vi "OfeliaPressure.vi"() -> ()   [LabVIEW 2017]
uses:
  <vilib>/Platform/TimedLoop/XDataNode/timing_clust.ctl
  <vilib>/Platform/TimedLoop/XDataNode/nitl_modes.ctl
  <vilib>/Platform/TimedLoop/XDataNode/wakeup.ctl
  <vilib>/Instr/_visa.llb/VISA Configure Serial Port (Instr).vi
  <vilib>/platform/TimedLoop/XDataNode/XDataNode.xnode
  <vilib>/Platform/TimedLoop/XDataNode/XDNodeRunTimeDep.lvlib
panel:
  in  "Initial":dbl
  in  "Period":i64
  out "Final Pressure S":dbl
  out "In Range?":bool
  in  "T-Ramp\nTarget Pressure (Bar) S":dbl=0.01
  out "error out 5":errorcluster
  in  "T-Ramp Slow":bool
  out "Waveform Chart":dbl(graph)
  out "Final Pressure":dbl
  in  "S-Ramps\nTarget Pressure (Bar)":dbl
  in  "T-Ramp":bool
  in  "S-Ramp":bool
  out "error out 4":errorcluster
  out "In Range?":bool
  out "error out 3":errorcluster
  in  "ZERO":bool
  out "Final Pressure":dbl
  out "Ramp Rate\nFinal Value":dbl
  out "In Range?":bool
  in  "T-Ramp\nTarget Pressure (Bar)":dbl=0.01
  out "error out 2":errorcluster
  in  "Step 2":bool
  out "In Range?":bool
  in  "Ramp Rate":dbl=0.01
  in  "Step 1":bool
  in  "Stop":bool
  in  "VISA resource name":refnum<visa-resource-name>="COM1"
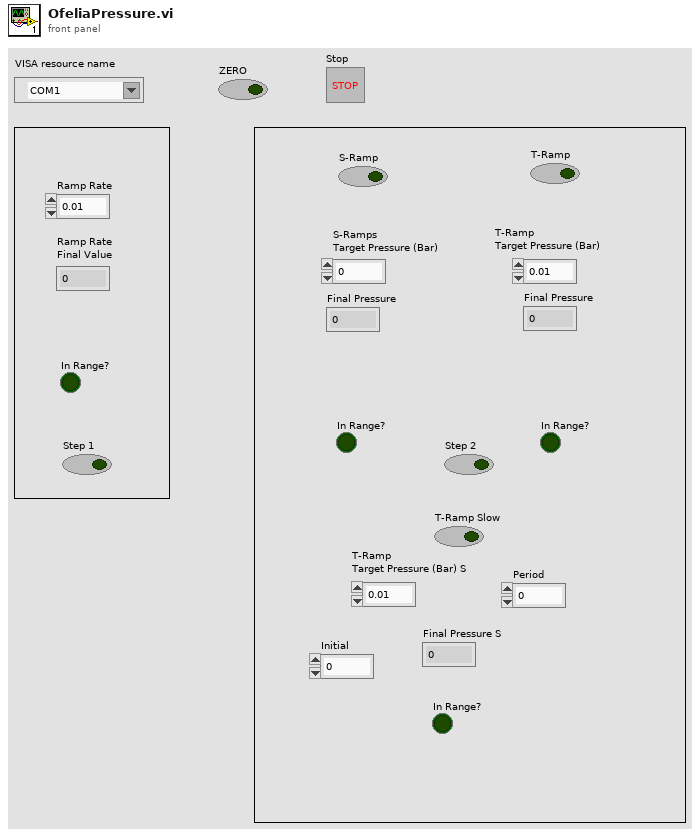
[diagram p1: front panel]
types:
  T1 = typedef "XDNodeRunTimeDep.lvlib/timing_clust.ctl" = cluster{"Expected End [f-1]":u64, "Actual End [f-1]":u64, "Finished Late? [f-1]":bool, "Expected End [i-1]":u64, "Actual End [i-1]":u64, "Finished Late? [i-1]":bool, "Expected Start [i]":u64, "Actual Start [i]":u64, "Expected Start [f]":u64, "Actual Start [f]":u64, "Source Name":string, "Structure Name":string, "Period":i64, "Deadline":i64, "Offset":i64, "Start":i64, "Priority":i32, "Timeout":i32, "Mode":T2, "Wakeup Reason":T3, "Error":errorcluster, "Source Type":string, "Secondary Source Type":string, "Global End Time":u64, "Global Start Time":u64, "Frame Duration":u64, "Iteration Duration":u64, "Assigned CPU":i32, "I/O Scan Engine Mode":u32}
  T2 = typedef "XDNodeRunTimeDep.lvlib/nitl_modes.ctl" = enum32{"No Change", "Process missed periods, maintain original phase", "Discard missed periods, maintain original phase", "Process missed periods, ignore original phase", "Discard missed periods, ignore original phase"}
  T3 = typedef "XDNodeRunTimeDep.lvlib/wakeup.ctl" = enum32{"Normal", "Aborted", "Asynchronous wakeup", "Timing source error", "Timed loop error", "Timeout"}
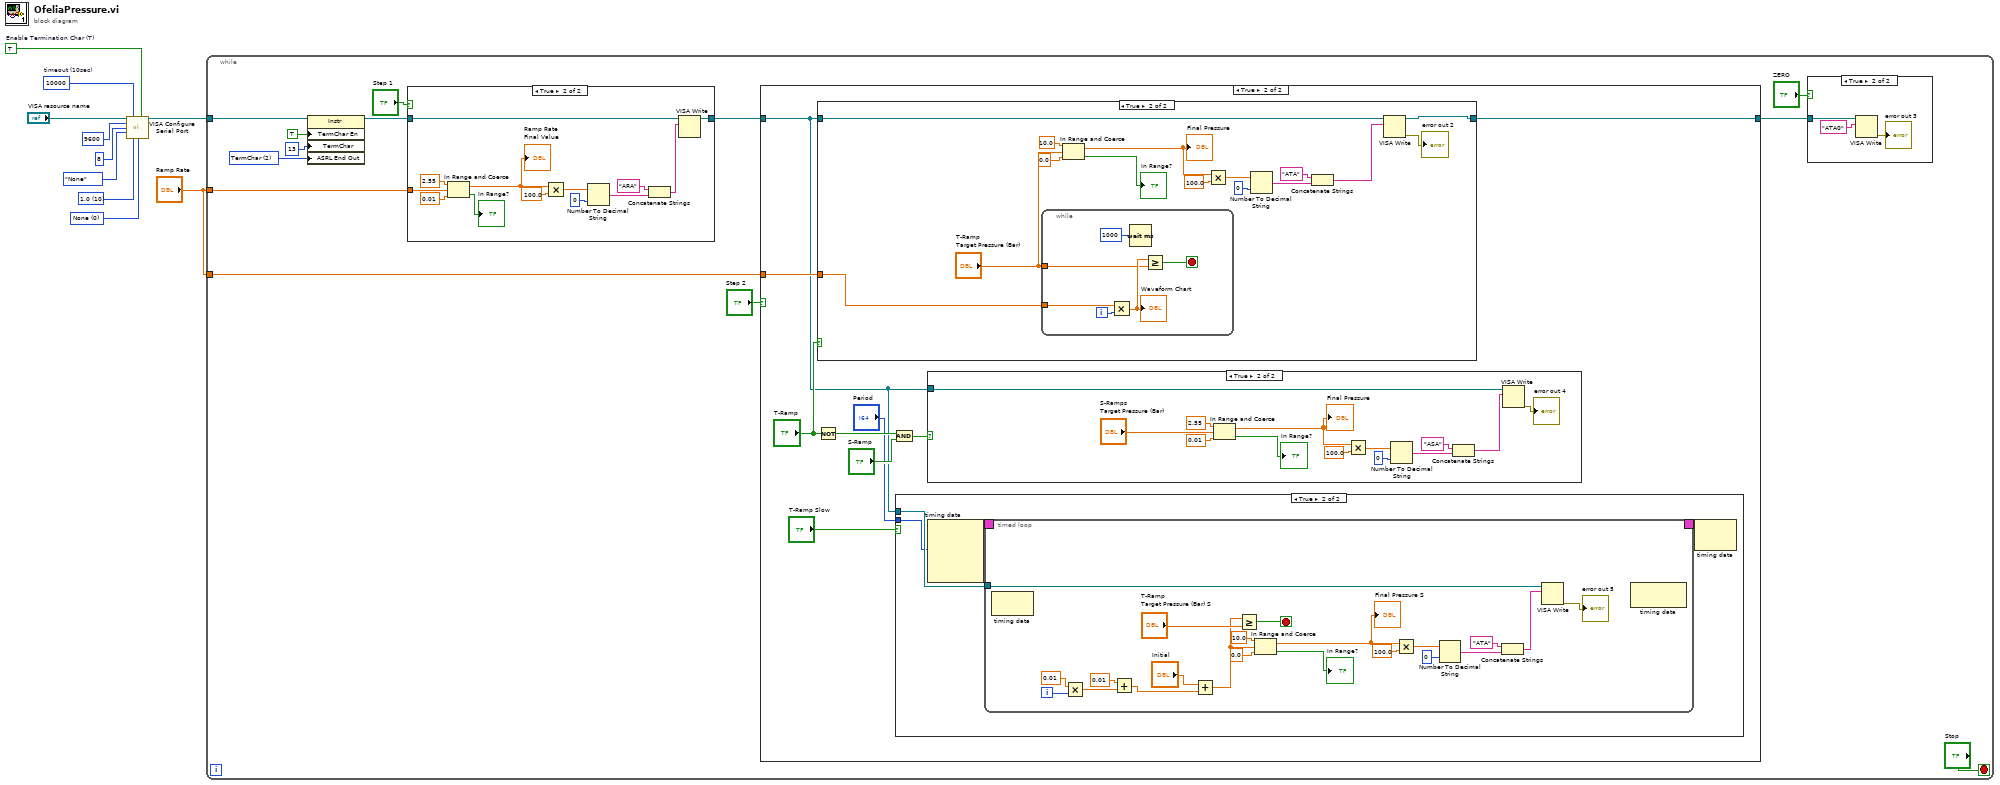
[diagram p0: block diagram]
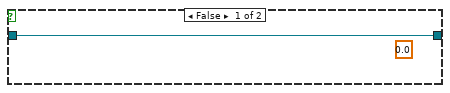
[diagram p7: hidden frame]
diagram:
  w7 = u16 10 items=["1.0"=10, "1.5"=15, "2.0"=20] ("stop bits")
  w2 = u16 0 items=["None"=0, "XON/XOFF"=1, "RTS/CTS"=2, "DTR/DSR"=4] ("flow control")
  w8 = TRUE  # Enable Termination Char (T)
  w9 = u32 10000  # timeout (10sec)
  n1 = call-poly "VISA Configure Serial Port"("VISA resource name"="VISA resource name", "timeout (10sec)"=w9, "Enable Termination\nChar (T)"=w8, "baud rate (9600)"=u32 9600 ("baud rate"), "data bits (8)"=u16 8 ("data bits"), "parity (0:none)"=enum16{"None", "Odd", "Even", "Mark", "Space"}."None", "stop bits (10: 1 bit)"=w7, "flow control (0:none)"=w2) -> ("VISA resource name out"=w3:refnum<visa-resource-name>)  [unwired: 1 in, 6 out]
  n2 = while {
    tunnel: w3 -> [w18]
    tunnel: "Ramp Rate" -> [w12]
    tunnel: "Ramp Rate" -> [w11]
    stop <- "Stop" stop-if-true
    w19 = u16 2 items=["None", "Last Bit", "TermChar", "Break"] ("Serial Settings:End Mode for Writes")
    n3 = property class="Instr"(reference=w18, "TermChar En"=TRUE ("Message Based Settings:Termination Character Enable"), "TermChar"=u8 13 ("Message Based Settings:Termination Character"), "ASRL End Out"=w19) -> (reference out=w17:refnum<visa-resource-name>)  [unwired: 1 in, 1 out]
    n4 = case shown="True" "Step 1" {
      tunnel: w17 -> [w103 w116]
      tunnel: [w103 w115] -> w15
      tunnel: w11 -> [_ w104]
      frame False {
        (unwired) 0.0 ("Ramp Rate")
      }
      frame True {
        n5 = In Range and Coerce(upper limit=2.55, x=w104, lower limit=0.01) -> (coerced(x)=w106:dbl, In Range?=→"In Range?":bool)
        "Ramp Rate\nFinal Value" <- w106
        n6 = Multiply(x=w106, y=100.0) -> (x*y=w107:dbl)
        n7 = Number To Decimal String(number=w107, width (-)=i16 0) -> (decimal integer string=w112:string)
        n8 = Concatenate Strings("ARA" ("write buffer"), w112) -> (w105:string)
        n9 = VISA Write(VISA resource name=w116, write buffer=w105) -> (VISA resource name out=w115:refnum<visa-resource-name>)  [unwired: 1 in, 2 out]
      }
    }
    n10 = case shown="True" "Step 2" {
      tunnel: w15 -> [w27 w29]
      tunnel: [w27 w36] -> w13
      tunnel: w12 -> [_ w31]
      frame False {
      }
      frame True {
        n11 = case shown="True" "T-Ramp" {
          tunnel: w29 -> [w81 w85]
          tunnel: [w81 w84] -> w36
          tunnel: w31 -> [_ w83]
          frame False {
          }
          frame True {
            n12 = while {
              tunnel: w83 -> [w102]
              tunnel: "T-Ramp\nTarget Pressure (Bar)" -> [w99]
              i -> [w101]
              stop <- w98 stop-if-true
              n13 = Multiply(x=w102, y=w101) -> (x*y=w100:dbl)
              "Waveform Chart" <- w100
              n14 = Wait (ms)(milliseconds to wait=u32 1000) -> ()  [unwired: 1 out]
              n15 = Greater Or Equal?(x=w100, y=w99) -> (x >= y?=w98:bool)
            }
            n16 = In Range and Coerce(upper limit=10.0, x="T-Ramp\nTarget Pressure (Bar)", lower limit=0.0) -> (coerced(x)=w88:dbl, In Range?=→"In Range?":bool)
            "Final Pressure" <- w88
            n17 = Multiply(x=w88, y=100.0) -> (x*y=w86:dbl)
            n18 = Number To Decimal String(number=w86, width (-)=i16 0) -> (decimal integer string=w92:string)
            n19 = Concatenate Strings("ATA" ("write buffer"), w92) -> (w94:string)
            n20 = VISA Write(VISA resource name=w85, write buffer=w94) -> (VISA resource name out=w84:refnum<visa-resource-name>, error out=→"error out 2":errorcluster)  [unwired: 1 in, 1 out]
          }
        }
        n21 = Not(x="T-Ramp") -> (.not. x?=w35:bool)
        n22 = And(x=w35, y="S-Ramp") -> (x .and. y?=w34:bool)
        n23 = case shown="True" "T-Ramp Slow" {
          tunnel: w29 -> [_ w38]
          tunnel: "Period" -> [_ w37]
          frame False {
          }
          frame True {
            n24 = node-c288(w37) -> (w40:T1)  [unwired: 3 in]
            n25 = timed-loop {
              timing: w40 -> [_]
              timing-out: [_] -> w39
              tunnel: w38 -> [w50]
              i -> [w48]
              stop <- w44 stop-if-true
              n26 = node-c288() -> ()  [unwired: 1 in, 1 out]
              n27 = Multiply(x=0.01 ("y"), y=w48) -> (x*y=w46:dbl)
              n28 = Add(x=0.01, y=w46) -> (x+y=w43:dbl)
              n29 = Add(x="Initial", y=w43) -> (x+y=w41:dbl)
              n30 = Greater Or Equal?(x=w41, y="T-Ramp\nTarget Pressure (Bar) S") -> (x >= y?=w44:bool)
              n31 = In Range and Coerce(upper limit=10.0, x=w41, lower limit=0.0) -> (coerced(x)=w53:dbl, In Range?=→"In Range?":bool)
              "Final Pressure S" <- w53
              n32 = Multiply(x=w53, y=100.0) -> (x*y=w51:dbl)
              n33 = Number To Decimal String(number=w51, width (-)=i16 0) -> (decimal integer string=w57:string)
              n34 = Concatenate Strings("ATA" ("write buffer"), w57) -> (w59:string)
              n35 = VISA Write(VISA resource name=w50, write buffer=w59) -> (error out=→"error out 5":errorcluster)  [unwired: 1 in, 2 out]
              n36 = node-c288() -> ()  [unwired: 1 in, 1 out]
            }
            n37 = node-c288(w39) -> ()  [unwired: 1 out]
          }
        }
        n38 = case shown="True" w34 {
          tunnel: w29 -> [_ w80]
          frame False {
          }
          frame True {
            n39 = In Range and Coerce(upper limit=2.55, x="S-Ramps\nTarget Pressure (Bar)", lower limit=0.01) -> (coerced(x)=w68:dbl, In Range?=→"In Range?":bool)
            "Final Pressure" <- w68
            n40 = Multiply(x=w68, y=100.0) -> (x*y=w71:dbl)
            n41 = Number To Decimal String(number=w71, width (-)=i16 0) -> (decimal integer string=w75:string)
            n42 = Concatenate Strings("ASA" ("write buffer"), w75) -> (w77:string)
            n43 = VISA Write(VISA resource name=w80, write buffer=w77) -> (error out=→"error out 4":errorcluster)  [unwired: 1 in, 2 out]
          }
        }
      }
    }
    n44 = case shown="True" "ZERO" {
      tunnel: w13 -> [_ w25]
      frame False {
      }
      frame True {
        n45 = VISA Write(VISA resource name=w25, write buffer="ATA0") -> (error out=→"error out 3":errorcluster)  [unwired: 1 in, 2 out]
      }
    }
  }
